vi "Append Element To Document.vi"(7 "Document in":refnum<class "xwpfDocument.lvclass">, 8 "error in (no error)":errorcluster, 11 "xwpfDocument.Element in":refnum<class "xwpfDocument.Element.lvclass">) -> (0 "error out":errorcluster, 3 "xwpfDocument.Element out":refnum<class "xwpfDocument.Element.lvclass">, 5 "Document out":refnum<class "xwpfDocument.lvclass">)   [LabVIEW 2017, in "Word_Specific.lvlib" / "xwpfDocument.Element.lvclass"]
uses:
  xwpfDocument.Element.lvclass
  xwpfDocument/xwpfDocument.lvclass
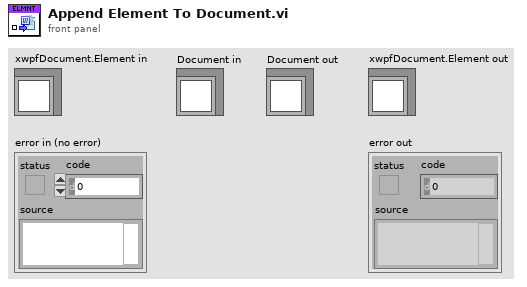
[diagram p1: front panel]
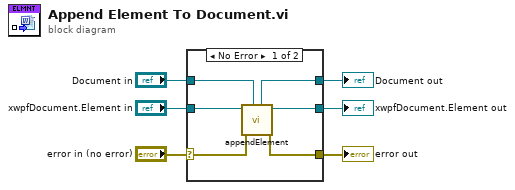
[diagram p0: block diagram]
diagram:
  n1 = case shown="No Error" "error in (no error)" {
    selector: "error in (no error)" -> [w11 w15]
    tunnel: [w10 w15] -> w5
    tunnel: [w9 w14] -> w3
    tunnel: "xwpfDocument.Element in" -> [w12 w14]
    tunnel: "Document in" -> [w8 w13]
    tunnel: [w7 w13] -> w1
    frame No Error {
      n2 = call-dynamic "appendElement.vi"("Document in"=w8, "error in (no error)"=w11, "xwpfDocument.Element in"=w12) -> ("error out"=w10:errorcluster, "xwpfDocument.Element out"=w9:refnum<class "xwpfDocument.Element.lvclass">, "Document out"=w7:refnum<class "xwpfDocument.lvclass">)  [unwired: 6 in]
    }
    frame Error {
    }
  }
  "error out" <- w5
  "xwpfDocument.Element out" <- w3
  "Document out" <- w1
